vi "Sine-Squared Ramp.vi"(7 "Samples":i32) -> (8 "Sine-squared ramp":dbl[](array[numeric]))   [LabVIEW 2020, in "Gate.lvclass"]
uses:
  Gate.lvclass
  <vilib>/Analysis/NI_AALBase.lvlib
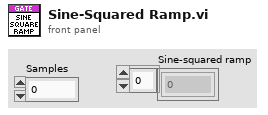
[diagram p1: front panel]
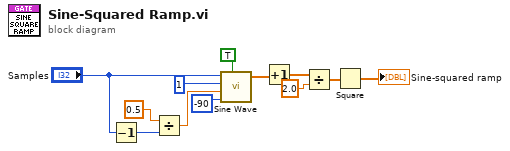
[diagram p0: block diagram]
diagram:
  n1 = Decrement(x="Samples") -> (x-1=w7:i32)
  n2 = Divide(x=0.5, y=w7) -> (x/y=w4:dbl)
  n3 = call <vilib>:"Sine Wave.vi"("samples"="Samples", "amplitude"=1, "frequency"=w4, "phase in"=-90, "reset phase"=TRUE) -> ("sine wave"=w9:dbl[])  [unwired: 2 out]
  n4 = Increment(x=w9) -> (x+1=w10:dbl[])
  n5 = Divide(x=w10, y=2.0) -> (x/y=w12:dbl[])
  n6 = Square(x=w12) -> (x^2=→"Sine-squared ramp":dbl[])
